vi "treat message.vi"(8 "error in (no error)":errorcluster, 11 "Roda_Filtros in":refnum<class "Roda_Filtros.lvclass">) -> (0 "error out":errorcluster, 2 "filter positioned":bool, 3 "Roda_Filtros out":refnum<class "Roda_Filtros.lvclass">)   [LabVIEW 2018, in "Roda_Filtros.lvclass"]
uses:
  Roda_Filtros.lvclass
  Roda_Filtros.lvclass/Roda_Filtros.ctl
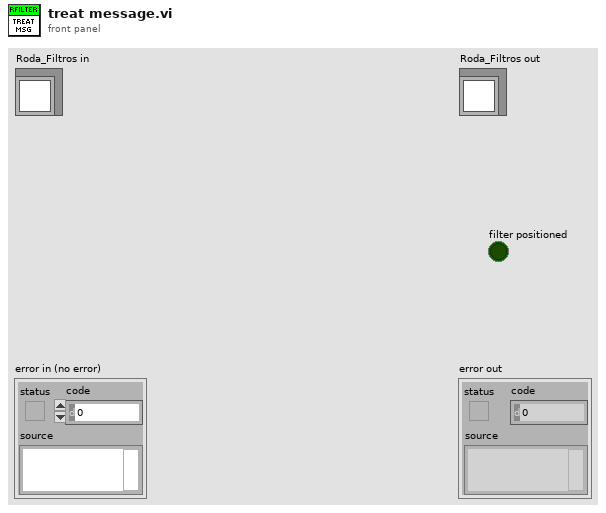
[diagram p1: front panel]
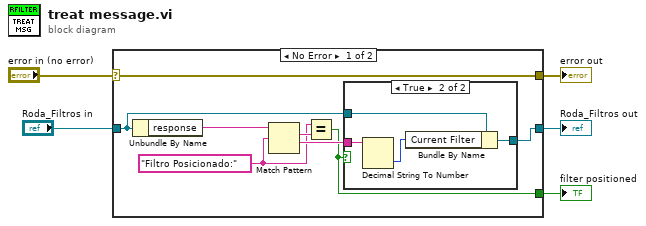
[diagram p0: block diagram]
diagram:
  n1 = case shown="No Error" "error in (no error)" {
    selector: "error in (no error)" -> [w13 w20]
    tunnel: [w13 w20] -> w4
    tunnel: [w9 w19] -> w2
    tunnel: "Roda_Filtros in" -> [w10 w19]
    tunnel: [w6 _] -> w1
    frame No Error {
      w7 = "Filtro Posicionado:"
      n2 = Unbundle By Name(w10) -> ("response"=w11:string)
      n3 = Match Pattern(string=w11, regular expression=w7) -> (match substring=w8:string, after substring=w12:string)  [unwired: 1 in, 2 out]
      n4 = Equal?(x=w7, y=w8) -> (x = y?=w6:bool)
      n5 = case shown="True" w6 {
        tunnel: w12 -> [_ w18]
        tunnel: w10 -> [w14 w17]
        tunnel: [w14 w16] -> w9
        frame False {
        }
        frame True {
          n6 = Decimal String To Number(string=w18) -> (number=w15:i32)  [unwired: 2 in, 1 out]
          n7 = Bundle By Name(cluster=w17, "Current Filter"=w15) -> (w16:refnum<class "Roda_Filtros.lvclass">)
        }
      }
    }
    frame Error {
    }
  }
  "error out" <- w4
  "Roda_Filtros out" <- w2
  "filter positioned" <- w1
